vi "Create Trial Params.vi"(11 "Function":string) -> (3 "Matlab Param Array":cluster{"Name":string, "Data":variant}[](array[cluster]))   [LabVIEW 2010]
panel:
  in  "matlabRandomization":bool
  in  "feedback":bool
  in  "fixSpot":bool
  in  "showColorTarget":bool
  in  "showGratingTarget":bool=TRUE
  in  "speed":i32(slide)=10 scale=0.0..10.0
  in  "rewardAmount":dbl=150.0
  in  "pAL":dbl(slide) scale=0.0..1.0
  in  "pA":dbl(slide)=0.5050505050505051 scale=0.0..1.0
  in  "cueTime":dbl=3000.0
  in  "targetTime":dbl=3000.0
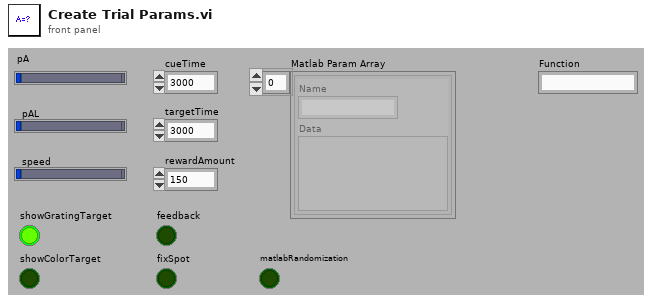
[diagram p1: front panel]
types:
  T1 = cluster{"Label.Text":string, "Variant":variant}[]
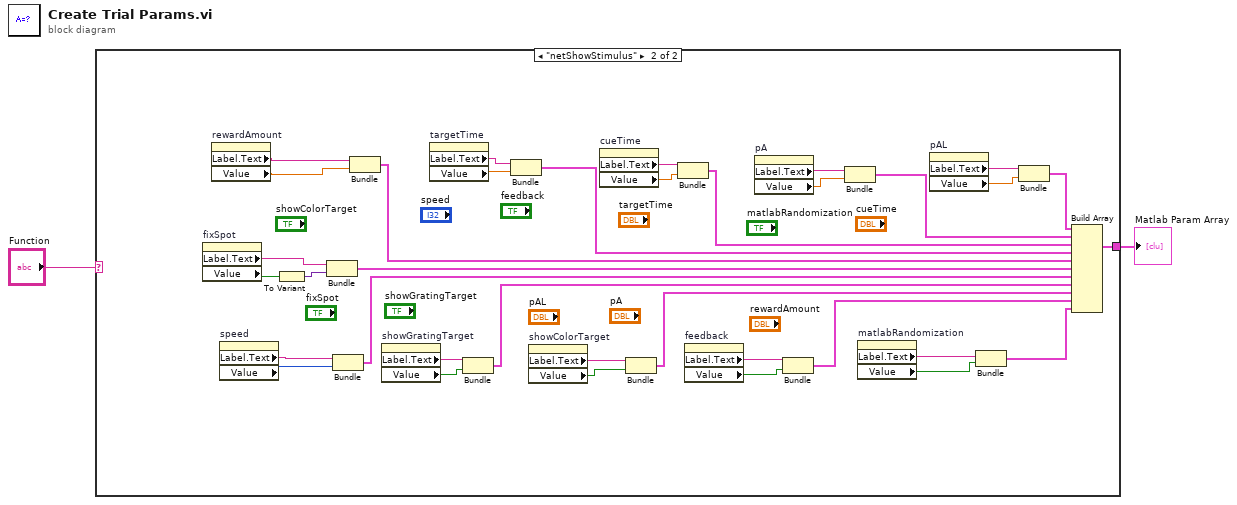
[diagram p0: block diagram]
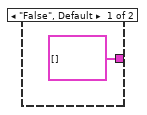
[diagram p2: hidden frame]
diagram:
  n1 = case shown="\"netShowStimulus\"" "Function" {
    tunnel: [T1 [] w25] -> w2
    frame "False", Default {
    }
    frame "netShowStimulus" {
      n2 = property on="fixSpot" class="Bool (strict)"() -> ("Label.Text"=w22:string, "Value"=w18:bool)  [unwired: 2 in, 2 out]
      n3 = property on="rewardAmount" class="DigNum (strict)"() -> ("Label.Text"=w24:string, "Value"=w23:dbl)  [unwired: 2 in, 2 out]
      n4 = property on="speed" class="Slide (strict)"() -> ("Label.Text"=w20:string, "Value"=w19:i32)  [unwired: 2 in, 2 out]
      n5 = To Variant(anything=w18) -> (Variant=w17:variant)
      n6 = Bundle("Label.Text"=w22, "Variant"=w17) -> (w21:cluster{"Label.Text":string, "Variant":variant})  [unwired: 1 in]
      n7 = Bundle("Label.Text"=w20, "Value"=w19) -> (w12:cluster{"Label.Text":string, "Value":i32})  [unwired: 1 in]
      n8 = Bundle("Label.Text"=w24, "Value"=w23) -> (w26:cluster{"Label.Text":string, "Value":dbl})  [unwired: 1 in]
      n9 = property on="showGratingTarget" class="Bool (strict)"() -> ("Label.Text"=w16:string, "Value"=w15:bool)  [unwired: 2 in, 2 out]
      n10 = property on="targetTime" class="DigNum (strict)"() -> ("Label.Text"=w38:string, "Value"=w37:dbl)  [unwired: 2 in, 2 out]
      n11 = Bundle("Label.Text"=w16, "Value"=w15) -> (w11:cluster{"Label.Text":string, "Value":bool})  [unwired: 1 in]
      n12 = Bundle("Label.Text"=w38, "Value"=w37) -> (w27:cluster{"Label.Text":string, "Value":dbl})  [unwired: 1 in]
      n13 = property on="showColorTarget" class="Bool (strict)"() -> ("Label.Text"=w14:string, "Value"=w13:bool)  [unwired: 2 in, 2 out]
      n14 = property on="cueTime" class="DigNum (strict)"() -> ("Label.Text"=w36:string, "Value"=w35:dbl)  [unwired: 2 in, 2 out]
      n15 = Bundle("Label.Text"=w14, "Value"=w13) -> (w10:cluster{"Label.Text":string, "Value":bool})  [unwired: 1 in]
      n16 = Bundle("Label.Text"=w36, "Value"=w35) -> (w28:cluster{"Label.Text":string, "Value":dbl})  [unwired: 1 in]
      n17 = property on="feedback" class="Bool (strict)"() -> ("Label.Text"=w9:string, "Value"=w8:bool)  [unwired: 2 in, 2 out]
      n18 = property on="pA" class="Slide (strict)"() -> ("Label.Text"=w34:string, "Value"=w33:dbl)  [unwired: 2 in, 2 out]
      n19 = Bundle("Label.Text"=w9, "Value"=w8) -> (w7:cluster{"Label.Text":string, "Value":bool})  [unwired: 1 in]
      n20 = Bundle("Label.Text"=w34, "Value"=w33) -> (w29:cluster{"Label.Text":string, "Value":dbl})  [unwired: 1 in]
      n21 = property on="matlabRandomization" class="Bool (strict)"() -> ("Label.Text"=w6:string, "Value"=w5:bool)  [unwired: 2 in, 2 out]
      n22 = property on="pAL" class="Slide (strict)"() -> ("Label.Text"=w32:string, "Value"=w31:dbl)  [unwired: 2 in, 2 out]
      n23 = Bundle("Label.Text"=w6, "Value"=w5) -> (w4:cluster{"Label.Text":string, "Value":bool})  [unwired: 1 in]
      n24 = Bundle("Label.Text"=w32, "Value"=w31) -> (w30:cluster{"Label.Text":string, "Value":dbl})  [unwired: 1 in]
      n25 = Build Array(w30, w29, w28, w27, w26, w21, w12, w11, w10, w7, w4) -> (w25:T1)
    }
  }
  "Matlab Param Array" <- w2
